vi "WebTestComplete.vi"(8 "error in (no error)":errorcluster, 10 "TestComplete in":T1, 11 "client handle":T2 caption="客户端句柄") -> (0 "错误输出":errorcluster, 1 "success":bool, 2 "Message":string, 3 "client handle out":T2 caption="客户端句柄输出", 4 "output":string, 5 "input":string)   [LabVIEW 2017]
uses:
  <vilib>/httpClient/LabVIEWHTTPClient.lvlib
  <vilib>/httpClient/POSTBuffer.vi
  <vilib>/httpClient/ClientHandle.ctl
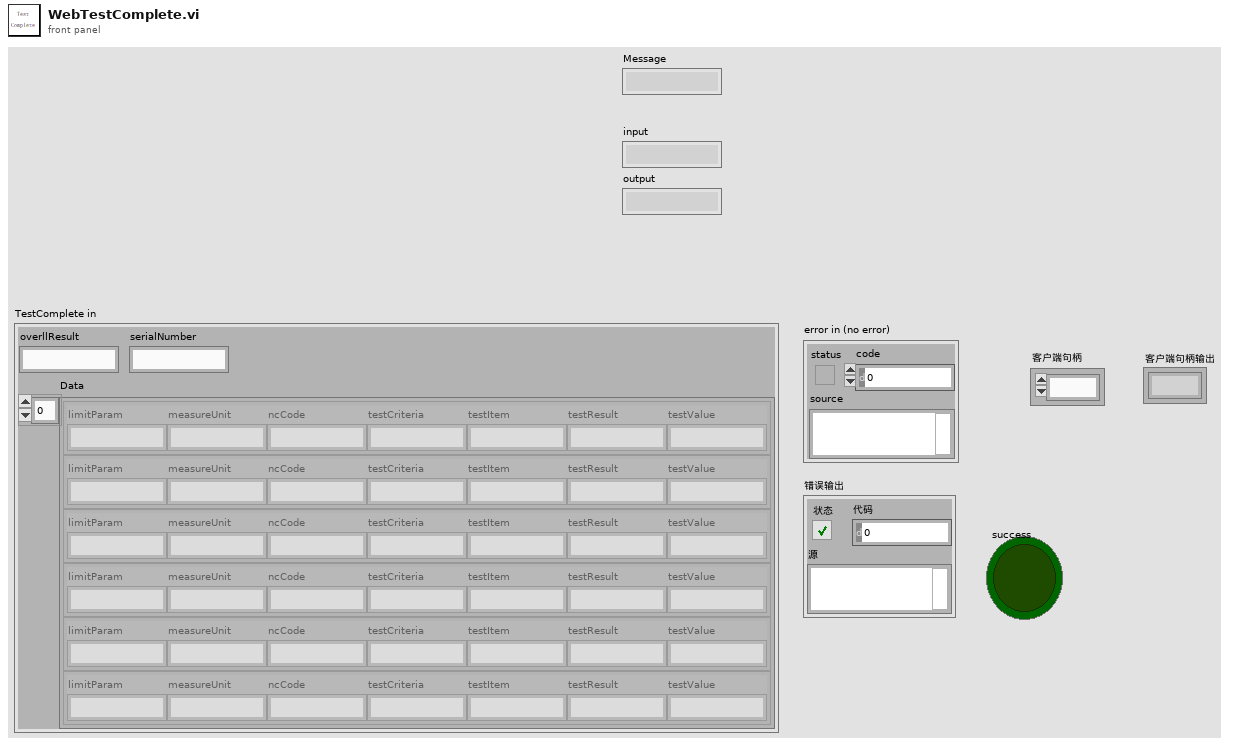
[diagram p1: front panel]
types:
  T1 = cluster{"overllResult":string, "serialNumber":string, "Data":cluster{"limitParam":string, "measureUnit":string, "ncCode":string, "testCriteria":string, "testItem":string, "testResult":string, "testValue":string}[]}
  T2 = typedef "LabVIEWHTTPClient.lvlib/ClientHandle.ctl" = refnum<k1>
  T3 = typedef "HD Config.ctl" = cluster{"ConnectPLC":cluster{"PLC Address":u8[], "PLC Port":i32, "PC Address":u8[]}, "FCO Model 4":cluster{"Com":refnum<visa-resource-name>, "Port":u32}, "FCO Model 7":cluster{"Com":refnum<visa-resource-name>, "Port":u32}, "Flow meter":cluster{"Com":refnum<visa-resource-name>, "Port":u32, "Units":enum16{"Standard", "Volumetric"}}}
  T4 = cluster{"limitParam":string, "measureUnit":string, "ncCode":string, "testCriteria":string, "testItem":string, "testResult":string, "testValue":string}[]
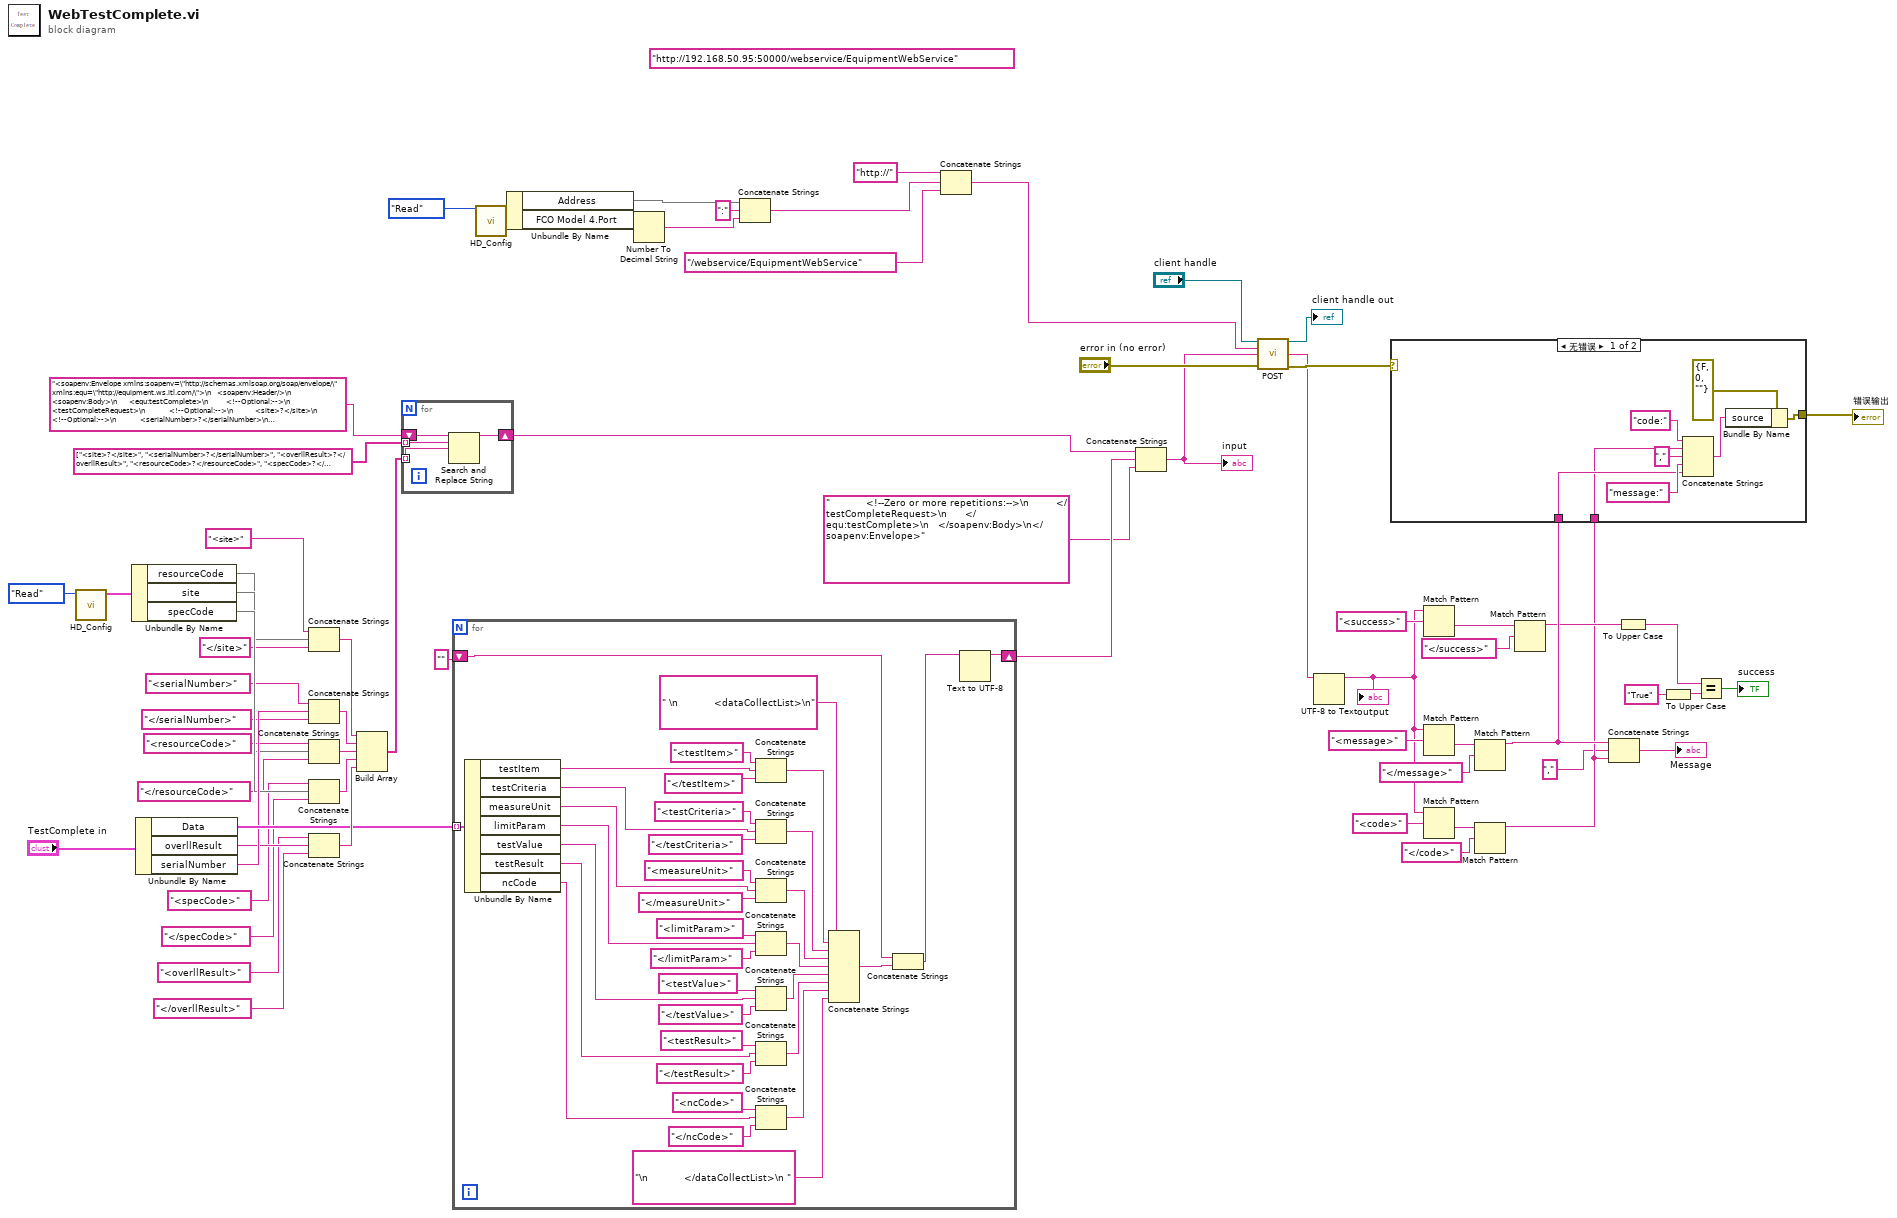
[diagram p0: block diagram]
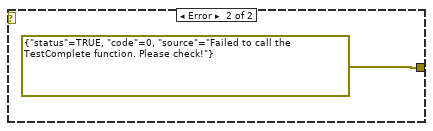
[diagram p2: hidden frame]
diagram:
  (unwired) "http://192.168.50.95:50000/webservice/EquipmentWebService" ("url")
  n1 = call "HD_Config.vi"("Step"=enum16{"Initial", "Write", "Read"}."Read") -> ("HD Config out"=w34:T3)  [unwired: 9 in, 1 out]
  n2 = Unbundle By Name(w34) -> ("resourceCode"=w27, "site"=w28, "specCode"=w29)
  n3 = Unbundle By Name("TestComplete in") -> ("Data"=w32:T4, "overllResult"=w30:string, "serialNumber"=w31:string)
  n4 = Concatenate Strings("<site>", w28, "</site>") -> (w40:string)
  n5 = Concatenate Strings("<serialNumber>", w31, "</serialNumber>") -> (w41:string)
  n6 = Concatenate Strings("<resourceCode>", w27, "</resourceCode>") -> (w42:string)
  n7 = Concatenate Strings("<specCode>", w29, "</specCode>") -> (w43:string)
  n8 = Concatenate Strings("<overllResult>", w30, "</overllResult>") -> (w44:string)
  n9 = Build Array(w40, w41, w42, w43, w44) -> (w45:string[])
  n10 = for {
    tunnel: string[] ["<site>?</site>", "<serialNumber>?</serialNumber>", "<overllResult>?</overllResult>", "<resourceCode>?</resourceCode>", "<specCode>?</specCode>"] -> [w71] mode=indexing
    tunnel: w45 -> [w70] mode=indexing
    shift-right: [w68] -> w38
    shift-left: "<soapenv:Envelope xmlns:soapenv=\"http://schemas.xmlsoap.org/soap/envelope/\" xmlns:equ=\"http://equipment.ws.itl.com/\">\n   <soapenv:Header/>\n   <soapenv:Body>\n      <equ:testComplete>\n         <!--Optional:-->\n         <testCompleteRequest>\n            <!--Optional:-->\n           <site>?</site>\n            <!--Optional:-->\n            <serialNumber>?</serialNumber>\n            <!--Optional:-->\n            <resourceCode>?</resourceCode>\n            <!--Optional:-->\n            <specCode>?</specCode>\n            <!--Optional:-->\n            <overllResult>?</overllResult>" -> [w69]
    n11 = Search and Replace String(input string=w69, search string=w71, replace string=w70) -> (result string=w68:string)  [unwired: 5 in, 3 out]
  }
  n12 = for {
    tunnel: w32 -> [w106] mode=indexing
    shift-right: [w77] -> w35
    shift-left: "" ("utf-8 text") -> [w74]
    n13 = Unbundle By Name(w106) -> ("testItem"=w84:string, "testCriteria"=w83:string, "measureUnit"=w82:string, "limitParam"=w81:string, "testValue"=w80:string, "testResult"=w79:string, "ncCode"=w78:string)
    n14 = Concatenate Strings("<testItem>", w84, "</testItem>") -> (w91:string)
    n15 = Concatenate Strings("<testCriteria>", w83, "</testCriteria>") -> (w90:string)
    n16 = Concatenate Strings("<measureUnit>", w82, "</measureUnit>") -> (w89:string)
    n17 = Concatenate Strings("<limitParam>", w81, "</limitParam>") -> (w88:string)
    n18 = Concatenate Strings("<testValue>", w80, "</testValue>") -> (w87:string)
    n19 = Concatenate Strings("<testResult>", w79, "</testResult>") -> (w86:string)
    n20 = Concatenate Strings("<ncCode>", w78, "</ncCode>") -> (w85:string)
    n21 = Concatenate Strings(" \n            <dataCollectList>\n" ("字符串"), w91, w90, w89, w88, w87, w86, w85, "\n            </dataCollectList>\n " ("字符串")) -> (w76:string)
    n22 = Concatenate Strings(w74, w76) -> (w75:string)
    n23 = Text to UTF-8(11:w75) -> (3:w77:string)  [unwired: 2 in, 1 out]
  }
  n24 = call "HD_Config.vi"("Step"=enum16{"Initial", "Write", "Read"}."Read") -> ("HD Config out"=w8:T3)  [unwired: 9 in, 1 out]
  n25 = Unbundle By Name(w8) -> ("Address"=w6, "FCO Model 4.Port"=w7:u32)
  n26 = Number To Decimal String(number=w7) -> (decimal integer string=w5:string)  [unwired: 1 in]
  n27 = Concatenate Strings(w6, ":" ("字符串"), w5) -> (w3:string)
  n28 = Concatenate Strings("http://" ("url"), w3, "/webservice/EquipmentWebService" ("url")) -> (w1:string)
  n29 = Concatenate Strings(w38, w35, "            <!--Zero or more repetitions:-->\n         </testCompleteRequest>\n      </equ:testComplete>\n   </soapenv:Body>\n</soapenv:Envelope>" ("字符串")) -> (w15:string)
  "input" <- w15
  n30 = call-poly <vilib>:"POST.vi"("client handle"="client handle", "url"=w1, "buffer"=w15, "error in (no error)"="error in (no error)") -> ("client handle out"=→"client handle out":T2, "body"=w54:string, "error out"=w65:errorcluster)  [unwired: 8 in, 1 out]
  n31 = UTF-8 to Text(11:w54) -> (3:w55:string)  [unwired: 2 in, 1 out]
  "output" <- w55
  n32 = Match Pattern(string=w55, regular expression="<success>") -> (after substring=w57:string)  [unwired: 1 in, 3 out]
  n33 = Match Pattern(string=w55, regular expression="<message>") -> (after substring=w60:string)  [unwired: 1 in, 3 out]
  n34 = Match Pattern(string=w55, regular expression="<code>") -> (after substring=w63:string)  [unwired: 1 in, 3 out]
  n35 = Match Pattern(string=w60, regular expression="</message>") -> (before substring=w53:string)  [unwired: 1 in, 3 out]
  n36 = Match Pattern(string=w63, regular expression="</code>") -> (before substring=w12:string)  [unwired: 1 in, 3 out]
  n37 = case shown="无错误" w65 {
    tunnel: [w109 errorcluster {"status"=TRUE, "code"=0, "source"="Failed to call the TestComplete function. Please check!"} ("error IO")] -> w48
    tunnel: w53 -> [w108 _]
    tunnel: w12 -> [w107 _]
    frame No Error {
      n38 = Concatenate Strings("code:" ("字符串"), w107, "," ("字符串"), "message:" ("字符串"), w108) -> (w111:string)
      n39 = Bundle By Name(cluster=errorcluster {"status"=FALSE, "code"=0, "source"=""} ("error IO"), "source"=w111) -> (w109:errorcluster)
    }
    frame Error {
    }
  }
  "错误输出" <- w48
  n40 = Match Pattern(string=w57, regular expression="</success>") -> (before substring=w51:string)  [unwired: 1 in, 3 out]
  n41 = Concatenate Strings(w53, "," ("string"), w12) -> (→"Message":string)
  n42 = To Upper Case(1:w51) -> (0:w50:string)
  n43 = To Upper Case(1:"True" ("子字符串之前")) -> (0:w49:string)
  n44 = Equal?(x=w50, y=w49) -> (x = y?=→"success":bool)
